vi "Auto Locate.vi"(1 "Autonomous?":bool, 2 "X from target":dbl) -> (0 "X Drive Arcade":dbl)   [LabVIEW 2012]
uses:
  BotStatus.vi
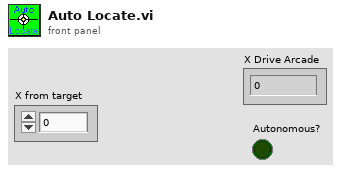
[diagram p1: front panel]
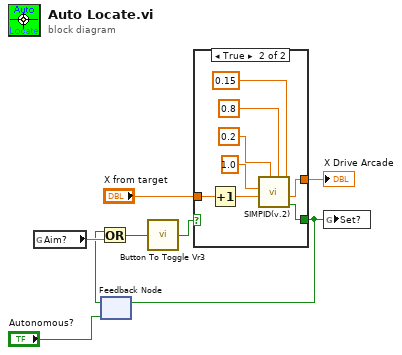
[diagram p0: block diagram]
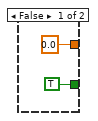
[diagram p2: hidden frame]
diagram:
  n1 = global read "BotStatus.vi" "Aim?"() -> (w7)
  n2 = feedback #1("Autonomous?") -> (w6:bool)
  n3 = Or(x=w6, y=w7) -> (x .or. y?=w8:bool)
  n4 = call "Button To Toggle Vr3.vi"("InValue"=w8) -> ("Result"=w1:bool)
  n5 = case shown="True" w1 {
    tunnel: [0.0 w13] -> w4
    tunnel: [TRUE ("On Target") w12] -> w3
    tunnel: "X from target" -> [_ w11]
    frame False {
    }
    frame True {
      n6 = Increment(x=w11) -> (x+1=w17:dbl)
      n7 = call "SIMPID(v.2).vi"("Range"=0.15, "upper limit"=0.8, "lower limit"=0.2, "Current Point"=w17, "Set Point"=1.0) -> ("On Target"=w12:bool, "result"=w13:dbl)  [unwired: 5 in]
    }
  }
  "X Drive Arcade" <- w4
  n8 = feedback-in #1(w3) -> ()
  n9 = global write "BotStatus.vi" "Set?"(w3) -> ()
